vi "Intensity Graph Linecut (Horizontal) (by val).vi"(6 "Averaging Method":enum16{"Step", "Gaussian"}(ring), 8 "error in (no error)":errorcluster, 9 "width (horizontal)":dbl, 10 "2D Data":dbl[][](array[numeric]), 11 "graph_utilities in":refnum<class "graph_utilities.lvclass">) -> (0 "error out":errorcluster, 2 "XY-data":cluster{"X-array":dbl[], "Y-array":dbl[]}[](array[cluster]), 3 "graph_utilities out":refnum<class "graph_utilities.lvclass">)   [LabVIEW 2019, in "graph_utilities.lvclass"]
doc: "Takes a Horizontal Linecut of an Intensity Graph and outputs to an XY Graph. The center location of the linecut is determined by the y-position of the Intensity Graph curser.\n - <b>width</b> is the standard deviation of a Gaussian function in the units of the Intensity Graph y scale.\n - If <b>width = 0 </b> the spacing between two adjacent data points will be used."
uses:
  graph_utilities.lvclass
  <vilib>/Analysis/NI_AALBase.lvlib
  <vilib>/Analysis/baseanly.llb/A x Vector.vi
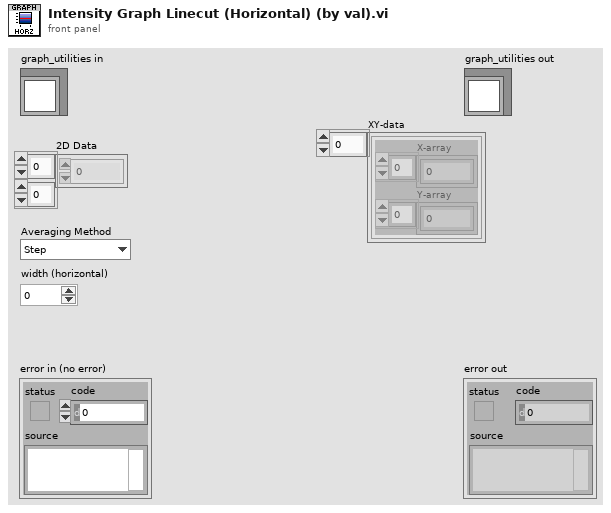
[diagram p1: front panel]
types:
  T1 = typedef "LVPointDoubleTypeDef.ctl" = cluster{"X":dbl, "Y":dbl}
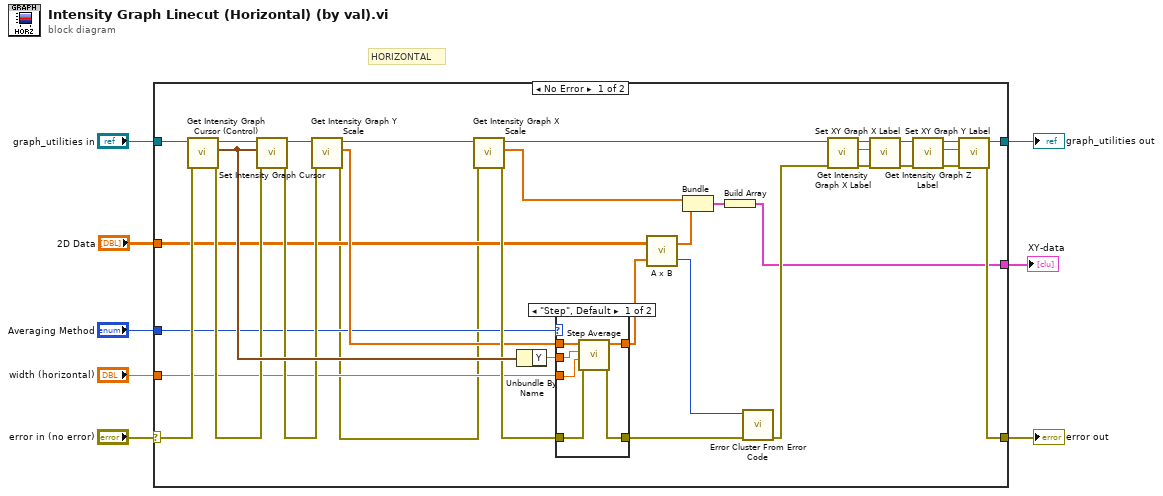
[diagram p0: block diagram]
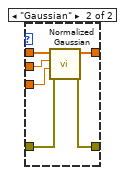
[diagram p2: hidden frame]
diagram:
  # "HORIZONTAL"
  n1 = case shown="No Error" "error in (no error)" {
    selector: "error in (no error)" -> [w33 w56]
    tunnel: [w14 w56] -> w7
    tunnel: [w18 w55] -> w5
    tunnel: "graph_utilities in" -> [w35 w55]
    tunnel: "width (horizontal)" -> [w21 _]
    tunnel: "Averaging Method" -> [w12 _]
    tunnel: "2D Data" -> [w11 _]
    tunnel: [w9 _] -> w1
    frame No Error {
      n2 = call "Get Intensity Graph Cursor (Control).vi"("error in (no error)"=w33, "graph_utilities in"=w35) -> ("error out"=w32:errorcluster, "Cursor.Cursor Position"=w37:T1, "graph_utilities out"=w36:refnum<class "graph_utilities.lvclass">)  [unwired: 7 in]
      n3 = call "Set Intensity Graph Cursor.vi"("error in (no error)"=w32, "Cursor.Cursor Position"=w37, "graph_utilities in"=w36) -> ("error out"=w31:errorcluster, "graph_utilities out"=w34:refnum<class "graph_utilities.lvclass">)  [unwired: 7 in]
      n4 = call "Get Intensity Graph Y Scale.vi"("error in (no error)"=w31, "graph_utilities in"=w34) -> ("error out"=w10:errorcluster, "Y Scale"=w22:dbl[], "graph_utilities out"=w38:refnum<class "graph_utilities.lvclass">)  [unwired: 6 in, 1 out]
      n5 = call "Get Intensity Graph X Scale.vi"("error in (no error)"=w10, "graph_utilities in"=w38) -> ("error out"=w30:errorcluster, "X Scale"=w39:dbl[], "graph_utilities out"=w23:refnum<class "graph_utilities.lvclass">)  [unwired: 6 in, 1 out]
      n6 = Unbundle By Name(w37) -> ("Y"=w41:dbl)
      n7 = case shown="\"Step\", Default" w12 {
        tunnel: [w45 w54] -> w42
        tunnel: w41 -> [w44 w53]
        tunnel: w30 -> [w47 w52]
        tunnel: [w46 w51] -> w29
        tunnel: w22 -> [w48 w50]
        tunnel: w21 -> [w43 w49]
        frame "Step", Default {
          n8 = call "Step Average.vi"("error in (no error)"=w47, "width (c)"=w43, "position (b)"=w44, "Scale"=w48) -> ("error out"=w46:errorcluster, "Averaged Result"=w45:dbl[])  [unwired: 4 in, 2 out]
        }
        frame "Gaussian" {
          n9 = call "Normalized Gaussian.vi"("error in (no error)"=w52, "width (c)"=w49, "position (b)"=w53, "Scale"=w50) -> ("error out"=w51:errorcluster, "Normalized Gaussian"=w54:dbl[])  [unwired: 6 in]
        }
      }
      n10 = call-poly <vilib>:"A x B.vi"("Vector"=w42, "A"=w11) -> ("error"=w40:i32, "A x Vector"=w13:dbl[])
      n11 = Bundle("X Scale"=w39, "A x Vector"=w13) -> (w28:cluster{"X Scale":dbl[], "A x Vector":dbl[]})  [unwired: 1 in]
      n12 = Build Array(w28) -> (w9:cluster{"X Scale":dbl[], "A x Vector":dbl[]}[])
      n13 = call <vilib>:"Error Cluster From Error Code.vi"("error in (no error)"=w29, "error code (0)"=w40) -> ("error out"=w27:errorcluster)  [unwired: 7 in]
      n14 = call "Get Intensity Graph X Label.vi"("error in (no error)"=w27, "graph_utilities in"=w23) -> ("error out"=w26:errorcluster, "X Label"=w24:string, "graph_utilities out"=w25:refnum<class "graph_utilities.lvclass">)  [unwired: 7 in]
      n15 = call "Set XY Graph X Label.vi"("error in (no error)"=w26, "X Label"=w24, "graph_utilities in"=w25) -> ("error out"=w16:errorcluster, "graph_utilities out"=w17:refnum<class "graph_utilities.lvclass">)  [unwired: 7 in]
      n16 = call "Get Intensity Graph Z Label.vi"("error in (no error)"=w16, "graph_utilities in"=w17) -> ("error out"=w15:errorcluster, "Z Label"=w20:string, "graph_utilities out"=w19:refnum<class "graph_utilities.lvclass">)  [unwired: 7 in]
      n17 = call "Set XY Graph Y Label.vi"("error in (no error)"=w15, "Y Label"=w20, "graph_utilities in"=w19) -> ("error out"=w14:errorcluster, "graph_utilities out"=w18:refnum<class "graph_utilities.lvclass">)  [unwired: 7 in]
    }
    frame Error {
    }
  }
  "error out" <- w7
  "graph_utilities out" <- w5
  "XY-data" <- w1
